vi "Build_Write File Record.vi"(0 "File Number":u16, 1 "Record Number":u16, 2 "values":u16[](array[numeric]), 3 "error in (no error)":errorcluster, 4 "仪器版本":T1) -> (7 "MB_PDU":T2={"Function Code"=1, "Data"=[], "RTU_DataBytes"=0}, 10 "error out":errorcluster)   [LabVIEW 2022 SP3, in "斯坦道氨氮.lvlib"]
uses:
  <vilib>/Plasmionique/MB Master/MB_PDU/MB_PDU_Cluster.ctl
  <vilib>/Plasmionique/MB Master/MB Master.lvlib
panel:
  out "添加的数组":u16[](array[numeric]) format="%x"
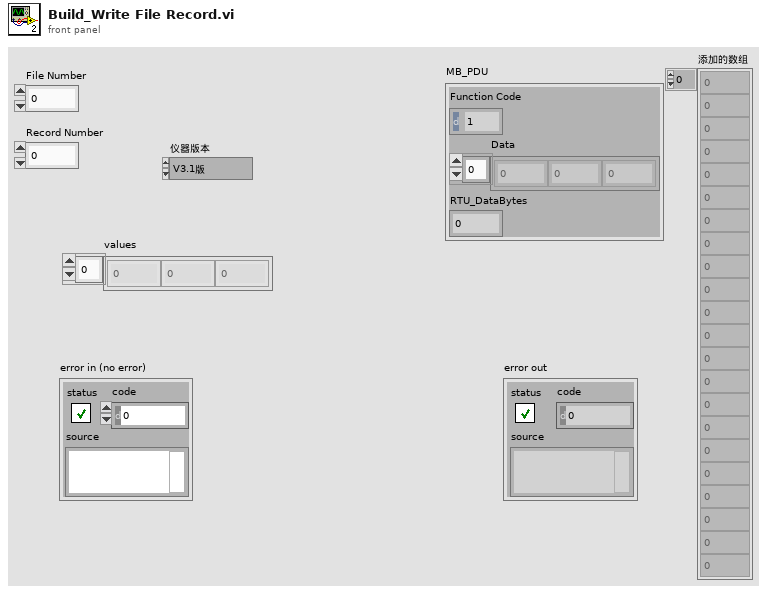
[diagram p1: front panel]
types:
  T1 = typedef "SingleStepTestV3.lvlib/SingleStepTestV3.lvclass/仪器版本.ctl" = enum16{"V3.1版", "V4版", "V3版", "V4.2版"}
  T2 = typedef "MB Master.lvlib/MB_PDU_Cluster.ctl" = cluster{"Function Code":u8, "Data":u8[], "RTU_DataBytes":i32}
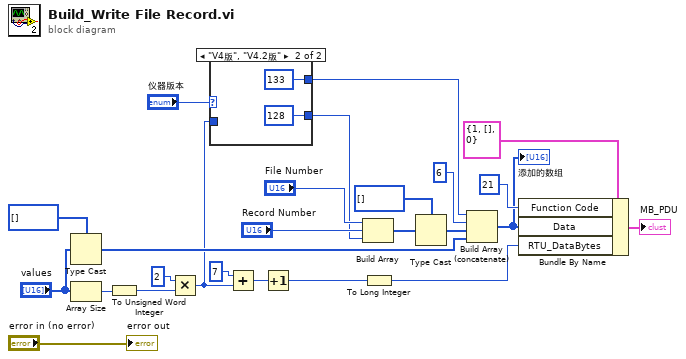
[diagram p0: block diagram]
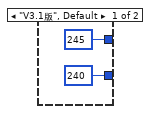
[diagram p2: hidden frame]
diagram:
  n1 = Type Cast(type=u8[] [], x="values") -> (*(type *) &x=w17:u8[])
  n2 = Array Size(array="values") -> (size(s)=w14:i32)
  n3 = To Unsigned Word Integer(number=w14) -> (unsigned 16bit integer=w5:u16)
  n4 = Multiply(x=u16 2, y=w5) -> (x*y=w1:u16)
  n5 = case shown="\"V4版\", \"V4.2版\"" "仪器版本" {
    tunnel: [u16 245 ("元素") u16 133 ("元素")] -> w3
    tunnel: [u16 240 ("元素") u16 128 ("元素")] -> w2
    tunnel: w1 -> [_ _]
    frame "V3.1版", Default {
    }
    frame "V4版", "V4.2版" {
    }
  }
  n6 = Add(x=u8 7, y=w1) -> (x+y=w9:u16)
  n7 = Increment(x=w9) -> (x+1=w8:u16)
  n8 = Build Array("File Number", "Record Number", w2) -> (w25:u16[])
  n9 = To Long Integer(number=w8) -> (32bit integer=w7:i32)
  n10 = Type Cast(type=u8[] [], x=w25) -> (*(type *) &x=w19:u8[])
  n11 = Build Array (concatenate)(w3, u8 6 ("元素"), w19, w17) -> (w16:u16[])
  "添加的数组" <- w16
  n12 = Bundle By Name(cluster=T2 {"Function Code"=1, "Data"=[], "RTU_DataBytes"=0} ("Modbus Serial New.lvlib:MB_PDU.lvclass"), "Function Code"=u8 21, "Data"=w16, "RTU_DataBytes"=w7) -> (→"MB_PDU":T2)
  "error out" <- "error in (no error)"
